vi "SLSC Search and Convert ENUM Value by Name.vi"(9 "enums":T1[](array[typedef]), 11 "Datatype Name":string) -> (1 "Enum":T1, 2 "Datatype found?":bool)   [LabVIEW 2017, in "SLSC Tree Control.lvlib"]
doc: "Search and convert a ENUM datatype based on the name of the item."
uses:
  SLSC Tree Control.lvlib
  Ctrl/Enum.ctl
  Ctrl/EnumValue.ctl
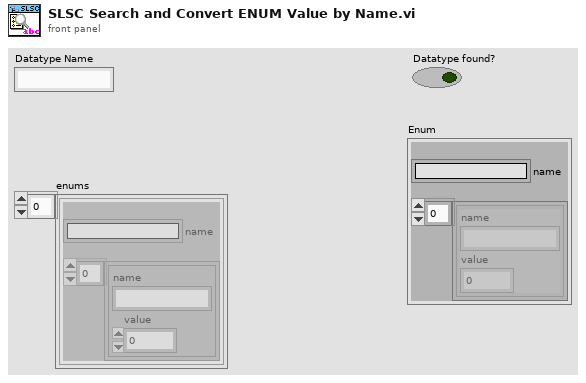
[diagram p1: front panel]
types:
  T1 = typedef "Enum.ctl" = cluster{"name":string, "values":T2[]}
  T2 = typedef "EnumValue.ctl" = cluster{"name":string, "value":i32}
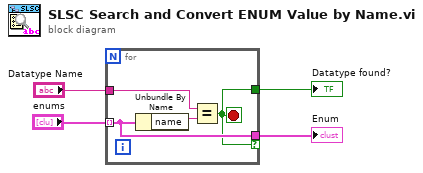
[diagram p0: block diagram]
diagram:
  n1 = for {
    tunnel: "enums" -> [w6] mode=indexing
    tunnel: "Datatype Name" -> [w7]
    tunnel: [w6] -> w2 if=w5
    tunnel: [w5] -> w3
    stop <- w5 stop-if-true
    n2 = Unbundle By Name(w6) -> ("name"=w8:string)
    n3 = Equal?(x=w7, y=w8) -> (x = y?=w5:bool)
  }
  "Datatype found?" <- w3
  "Enum" <- w2
